vi "Write and Get Channel Reading.vi"(8 "error in":errorcluster, 9 "Readings":digitalwaveform[](array[waveform]), 10 "Channel":string, 11 "Buffer Lossless Bin in":refnum<class "Buffer Lossless Digital.lvclass">) -> (0 "error out":errorcluster, 2 "Reading":digitalwaveform(waveform), 3 "Buffer Lossless Bin out":refnum<class "Buffer Lossless Digital.lvclass">)   [LabVIEW 2024, in "Buffer Lossless Digital.lvclass"]
uses:
  Buffer Lossless Digital.lvclass
  Buffer Lossless Digital.lvclass/Buffer Lossless Digital.ctl
  <vilib>/Waveform/DWDTOps.llb/DWDT Append Digital Samples.vi
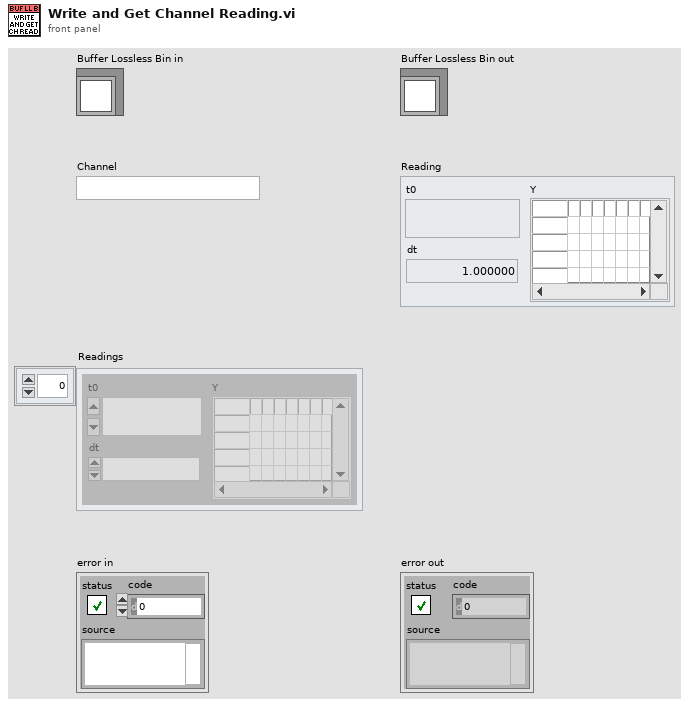
[diagram p1: front panel]
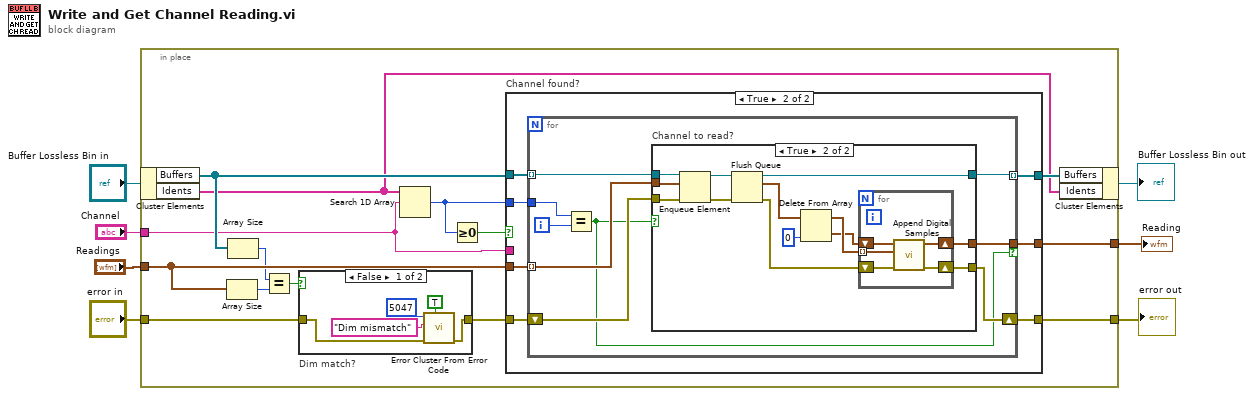
[diagram p0: block diagram]
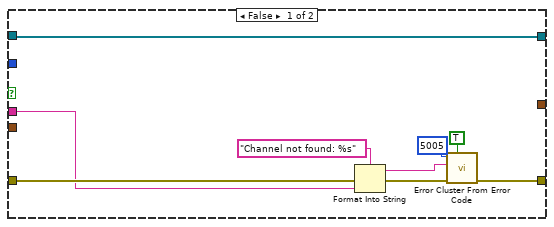
[diagram p3: hidden frame]
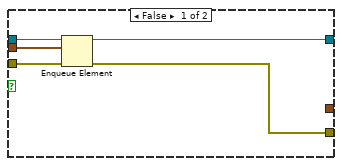
[diagram p4: hidden frame]
diagram:
  n1 = in-place {
    in-place-border: "Readings" -> [w18]
    in-place-border: "error in" -> [w13]
    in-place-border: [w21] -> w1
    in-place-border: "Channel" -> [w8]
    in-place-border: [w9] -> w3
    n2 = in-place-cluster #1("Buffer Lossless Bin in") -> ("Buffers"=w17:refnum<queue>[], "Idents"=w10:string[])
    n3 = Array Size(array=w18) -> (size(s)=w14:i32)
    n4 = Array Size(array=w17) -> (size(s)=w15:i32)
    n5 = Equal?(x=w15, y=w14) -> (x = y?=w16:bool)
    n6 = case "Dim match?" shown="False" w16 {
      tunnel: w13 -> [w26 w27]
      tunnel: [w25 w27] -> w12
      frame False {
        n7 = call <vilib>:"Error Cluster From Error Code.vi"("show call chain? (False)"=TRUE, "error in (no error)"=w26, "error message (\"\")"="Dim mismatch" ("error message (\"\")"), "error code (0)"=5047) -> ("error out"=w25:errorcluster)  [unwired: 5 in]
      }
      frame True {
      }
    }
    n8 = Search 1D Array(1D array=w10, element=w8) -> (index of element=w20:i32)  [unwired: 1 in]
    n9 = Greater Or Equal To 0?(x=w20) -> (x >= 0?=w19:bool)
    n10 = case "Channel found?" shown="True" w19 {
      tunnel: w12 -> [w31 w43]
      tunnel: [w30 w42] -> w21
      tunnel: w17 -> [w29 w39]
      tunnel: w20 -> [_ w41]
      tunnel: w18 -> [_ w40]
      tunnel: [w29 w38] -> w11
      tunnel: [_ w37] -> w9
      tunnel: w8 -> [w28 _]
      frame False {
        n11 = Format Into String(format string="Channel not found: %s", error in=w31, w28) -> (resulting string=w32:string, error out=w34:errorcluster)  [unwired: 1 in]
        n12 = call <vilib>:"Error Cluster From Error Code.vi"("show call chain? (False)"=TRUE, "error in (no error)"=w34, "error message (\"\")"=w32, "error code (0)"=5005) -> ("error out"=w30:errorcluster)  [unwired: 5 in]
      }
      frame True {
        n13 = for {
          tunnel: w41 -> [w48]
          shift-right: [w49] -> w42
          shift-left: w43 -> [w50]
          tunnel: w40 -> [w51] mode=indexing
          tunnel: w39 -> [w52] mode=indexing
          tunnel: [w46] -> w38 mode=indexing
          tunnel: [w45] -> w37 if=w44
          i -> [w47]
          n14 = Equal?(x=w48, y=w47) -> (x = y?=w44:bool)
          n15 = case "Channel to read?" shown="True" w44 {
            tunnel: w52 -> [w57 w67]
            tunnel: w51 -> [w53 w65]
            tunnel: w50 -> [w56 w69]
            tunnel: [w55 w62] -> w49
            tunnel: [w54 w70] -> w46
            tunnel: [_ w63] -> w45
            frame False {
              n16 = Enqueue Element(queue=w57, element=w53, error in (no error)=w56) -> (queue out=w54:refnum<queue>, error out=w55:errorcluster)  [unwired: 1 in, 1 out]
            }
            frame True {
              n17 = Enqueue Element(queue=w67, element=w65, error in (no error)=w69) -> (queue out=w66:refnum<queue>, error out=w68:errorcluster)  [unwired: 1 in, 1 out]
              n18 = Flush Queue(queue=w66, error in (no error)=w68) -> (queue out=w70:refnum<queue>, remaining elements=w61:digitalwaveform[], error out=w64:errorcluster)
              n19 = Delete From Array(array=w61, index=0) -> (deleted portion=w58:digitalwaveform, array with subset deleted=w59:digitalwaveform[])  [unwired: 1 in]
              n20 = for {
                tunnel: w59 -> [w72] mode=indexing
                shift-right: [w73] -> w63
                shift-left: w58 -> [w71]
                shift-right: [w74] -> w62
                shift-left: w64 -> [w75]
                n21 = call-poly <vilib>:"Append Digital Samples.vi"("error in (no error)"=w75, "digital waveform B"=w72, "digital waveform A"=w71) -> ("error out"=w74:errorcluster, "digital waveform out"=w73:digitalwaveform)  [unwired: 7 in]
              }
            }
          }
        }
      }
    }
    n22 = in-place-cluster #1("Buffers"=w11, "Idents"=w10) -> (→"Buffer Lossless Bin out":refnum<class "Buffer Lossless Digital.lvclass">)
  }
  "error out" <- w1
  "Reading" <- w3
